vi "Heater Main PID 3.vi"() -> ()   [LabVIEW 2019]
doc: "This example demonstrates how to acquire a continuous amount of data (Waveform) using the DAQ device's internal clock. It also shows how to synchronize two devices for different device families (E Series, S Series, M Series, X Series, DSA, and SC Express), to simultaneously acquire the data.\n\nFor instructions on how to connect your signals to the DAQ device, refer to your device documentation."
uses:
  <vilib>/Utility/error.llb/DialogType.ctl
  <vilib>/DAQmx/read.llb/DAQmx Read (Analog 1D Wfm NChan NSamp).vi
  <vilib>/DAQmx/write.llb/DAQmx Write (Analog DBL 1Chan 1Samp).vi
  <vilib>/DAQmx/create/channels.llb/DAQmx Create Channel (AO-Voltage-Basic).vi
  <vilib>/DAQmx/create/channels.llb/DAQmx Create Channel (AI-Voltage-Basic).vi
panel:
  in  "AI Channel - Heater Shunt":tag
  in  "Channel - Heater V":tag
  in  "Voltage":dbl=1.0 caption="Amplitude"
  in  "Channel config":T1
  in  "error in":errorcluster
  in  "task in":refnum<k21>
  in  "Microhotplate Logger":T2(tab)=enum."Heater config"
  in  "Stop":bool
  in  "Enable logging":bool caption="Enable"
  in  "File config":T3={"Filepath"=path "C:/Users/Administrator/Desktop/DAQ Heater Control/Test data", "Test ID"="test", "PC"="69DTQV2"}
  out "Logging":bool
  in  "Current channel config":T4={"Channel Index"=1, "Shunt resistance"=10.0, "Channel name"="Heater Current"} {"Shunt resistance" format="%.4f"}
  in  "IV channel config":T5={"Voltage channel index"=0, "Current channel index"=2}
  out "IV channel names":T6={"Voltage channel name"="Heater Voltage", "Current channel name"="Heater Current"}
  in  "TCR config":T7={"TCR1"=0.00205, "TCR2"=3e-07, "TRH"=0.766, "TRM"=0.928} {"TRM" format="%.3f"; "TRH" format="%.3f"; "TCR2" format="%.2e"; "TCR1" format="%.2e"}
  in  "Ramb config":cluster{"Tamb":dbl, "Ramb":dbl}={"Tamb"=25.0, "Ramb"=4.84} {"Ramb" format="%.3f"; "Tamb" format="%.3f"}
  out "Shunt channel name":string="Heater Shunt"
  out "PID output":dbl=1.0
  out "PID input":dbl
  in  "Setpoint":i32=2
  in  "Increment":dbl format="%.4f"
  out "Overrange":bool
  out "Heater shunt":dynamicdata(graph)=[{"t0"=timestamp(3680167673.7458043 s since 1904-01-01), "dt"=0.001, "Y"=[0.23414337637449473], "attributes"=variant("NI_ChannelName"=variant(string "Heater Voltage (DC Voltage)"), "NI_OriginalChannelName"=variant(string "Heater Voltage"), "NI_UnitDescription"=variant(string "Volts"))}, {"t0"=timestamp(3680167673.7458158 s since 1904-01-01), "dt"=0.001, "Y"=[0.4133136878458651], "attributes"=variant("NI_ChannelName"=variant(string "Heater Shunt (DC Voltage)"), "NI_OriginalChannelName"=variant(string "Heater Shunt"), "NI_UnitDescription"=variant(string "Volts"))}, {"t0"=timestamp(3680167673.7458158 s since 1904-01-01), "dt"=0.001, "Y"=[0.04133136878458673], "attributes"=variant("NI_ChannelName"=variant(string "Heater Current (DC Voltage)"), "NI_OriginalChannelName"=variant(string "Heater Current"), "NI_UnitDescription"=variant(string "A"))}, {"t0"=timestamp(3680167673.7458043 s since 1904-01-01), "dt"=0.001, "Y"=[5.665028733285053], "attributes"=variant("NI_ChannelName"=variant(string "Heater Resistance (DC Voltage)"), "NI_OriginalChannelName"=variant(string "Heater Resistance"), "NI_UnitDescription"=variant(string "Ohms"))}, {"t0"=timestamp(3680167673.7458043 s since 1904-01-01), "dt"=0.001, "Y"=[0.009677466447099818], "attributes"=variant("NI_ChannelName"=variant(string "Heater Power (DC Voltage)"), "NI_OriginalChannelName"=variant(string "Heater Power"), "NI_UnitDescription"=variant(string "Ohms"))}, {"t0"=timestamp(3680167673.7458043 s since 1904-01-01), "dt"=0.001, "Y"=[124.29416718343353], "attributes"=variant("NI_ChannelName"=variant(string "Heater Temp (DC Voltage)"), "NI_OriginalChannelName"=variant(string "Heater Temp"), "NI_UnitDescription"=variant(string "degC"))}]
  out "Heater temperature":dynamicdata(graph)=[{"t0"=timestamp(3680167673.7458043 s since 1904-01-01), "dt"=0.001, "Y"=[0.23414337637449473], "attributes"=variant("NI_ChannelName"=variant(string "Heater Voltage (DC Voltage)"), "NI_OriginalChannelName"=variant(string "Heater Voltage"), "NI_UnitDescription"=variant(string "Volts"))}, {"t0"=timestamp(3680167673.7458158 s since 1904-01-01), "dt"=0.001, "Y"=[0.4133136878458651], "attributes"=variant("NI_ChannelName"=variant(string "Heater Shunt (DC Voltage)"), "NI_OriginalChannelName"=variant(string "Heater Shunt"), "NI_UnitDescription"=variant(string "Volts"))}, {"t0"=timestamp(3680167673.7458158 s since 1904-01-01), "dt"=0.001, "Y"=[0.04133136878458673], "attributes"=variant("NI_ChannelName"=variant(string "Heater Current (DC Voltage)"), "NI_OriginalChannelName"=variant(string "Heater Current"), "NI_UnitDescription"=variant(string "A"))}, {"t0"=timestamp(3680167673.7458043 s since 1904-01-01), "dt"=0.001, "Y"=[5.665028733285053], "attributes"=variant("NI_ChannelName"=variant(string "Heater Resistance (DC Voltage)"), "NI_OriginalChannelName"=variant(string "Heater Resistance"), "NI_UnitDescription"=variant(string "Ohms"))}, {"t0"=timestamp(3680167673.7458043 s since 1904-01-01), "dt"=0.001, "Y"=[0.009677466447099818], "attributes"=variant("NI_ChannelName"=variant(string "Heater Power (DC Voltage)"), "NI_OriginalChannelName"=variant(string "Heater Power"), "NI_UnitDescription"=variant(string "Ohms"))}, {"t0"=timestamp(3680167673.7458043 s since 1904-01-01), "dt"=0.001, "Y"=[124.29416718343353], "attributes"=variant("NI_ChannelName"=variant(string "Heater Temp (DC Voltage)"), "NI_OriginalChannelName"=variant(string "Heater Temp"), "NI_UnitDescription"=variant(string "degC"))}]
  out "Heater current":dynamicdata(graph)=[{"t0"=timestamp(3680167673.7458043 s since 1904-01-01), "dt"=0.001, "Y"=[0.23414337637449473], "attributes"=variant("NI_ChannelName"=variant(string "Heater Voltage (DC Voltage)"), "NI_OriginalChannelName"=variant(string "Heater Voltage"), "NI_UnitDescription"=variant(string "Volts"))}, {"t0"=timestamp(3680167673.7458158 s since 1904-01-01), "dt"=0.001, "Y"=[0.4133136878458651], "attributes"=variant("NI_ChannelName"=variant(string "Heater Shunt (DC Voltage)"), "NI_OriginalChannelName"=variant(string "Heater Shunt"), "NI_UnitDescription"=variant(string "Volts"))}, {"t0"=timestamp(3680167673.7458158 s since 1904-01-01), "dt"=0.001, "Y"=[0.04133136878458673], "attributes"=variant("NI_ChannelName"=variant(string "Heater Current (DC Voltage)"), "NI_OriginalChannelName"=variant(string "Heater Current"), "NI_UnitDescription"=variant(string "A"))}, {"t0"=timestamp(3680167673.7458043 s since 1904-01-01), "dt"=0.001, "Y"=[5.665028733285053], "attributes"=variant("NI_ChannelName"=variant(string "Heater Resistance (DC Voltage)"), "NI_OriginalChannelName"=variant(string "Heater Resistance"), "NI_UnitDescription"=variant(string "Ohms"))}, {"t0"=timestamp(3680167673.7458043 s since 1904-01-01), "dt"=0.001, "Y"=[0.009677466447099818], "attributes"=variant("NI_ChannelName"=variant(string "Heater Power (DC Voltage)"), "NI_OriginalChannelName"=variant(string "Heater Power"), "NI_UnitDescription"=variant(string "Ohms"))}, {"t0"=timestamp(3680167673.7458043 s since 1904-01-01), "dt"=0.001, "Y"=[124.29416718343353], "attributes"=variant("NI_ChannelName"=variant(string "Heater Temp (DC Voltage)"), "NI_OriginalChannelName"=variant(string "Heater Temp"), "NI_UnitDescription"=variant(string "degC"))}]
  out "Heater voltage":dynamicdata(graph)=[{"t0"=timestamp(3680167673.7458043 s since 1904-01-01), "dt"=0.001, "Y"=[0.23414337637449473], "attributes"=variant("NI_ChannelName"=variant(string "Heater Voltage (DC Voltage)"), "NI_OriginalChannelName"=variant(string "Heater Voltage"), "NI_UnitDescription"=variant(string "Volts"))}, {"t0"=timestamp(3680167673.7458158 s since 1904-01-01), "dt"=0.001, "Y"=[0.4133136878458651], "attributes"=variant("NI_ChannelName"=variant(string "Heater Shunt (DC Voltage)"), "NI_OriginalChannelName"=variant(string "Heater Shunt"), "NI_UnitDescription"=variant(string "Volts"))}, {"t0"=timestamp(3680167673.7458158 s since 1904-01-01), "dt"=0.001, "Y"=[0.04133136878458673], "attributes"=variant("NI_ChannelName"=variant(string "Heater Current (DC Voltage)"), "NI_OriginalChannelName"=variant(string "Heater Current"), "NI_UnitDescription"=variant(string "A"))}, {"t0"=timestamp(3680167673.7458043 s since 1904-01-01), "dt"=0.001, "Y"=[5.665028733285053], "attributes"=variant("NI_ChannelName"=variant(string "Heater Resistance (DC Voltage)"), "NI_OriginalChannelName"=variant(string "Heater Resistance"), "NI_UnitDescription"=variant(string "Ohms"))}, {"t0"=timestamp(3680167673.7458043 s since 1904-01-01), "dt"=0.001, "Y"=[0.009677466447099818], "attributes"=variant("NI_ChannelName"=variant(string "Heater Power (DC Voltage)"), "NI_OriginalChannelName"=variant(string "Heater Power"), "NI_UnitDescription"=variant(string "Ohms"))}, {"t0"=timestamp(3680167673.7458043 s since 1904-01-01), "dt"=0.001, "Y"=[124.29416718343353], "attributes"=variant("NI_ChannelName"=variant(string "Heater Temp (DC Voltage)"), "NI_OriginalChannelName"=variant(string "Heater Temp"), "NI_UnitDescription"=variant(string "degC"))}]
  out "Heater resistance":dynamicdata(graph)=[{"t0"=timestamp(3680167673.7458043 s since 1904-01-01), "dt"=0.001, "Y"=[0.23414337637449473], "attributes"=variant("NI_ChannelName"=variant(string "Heater Voltage (DC Voltage)"), "NI_OriginalChannelName"=variant(string "Heater Voltage"), "NI_UnitDescription"=variant(string "Volts"))}, {"t0"=timestamp(3680167673.7458158 s since 1904-01-01), "dt"=0.001, "Y"=[0.4133136878458651], "attributes"=variant("NI_ChannelName"=variant(string "Heater Shunt (DC Voltage)"), "NI_OriginalChannelName"=variant(string "Heater Shunt"), "NI_UnitDescription"=variant(string "Volts"))}, {"t0"=timestamp(3680167673.7458158 s since 1904-01-01), "dt"=0.001, "Y"=[0.04133136878458673], "attributes"=variant("NI_ChannelName"=variant(string "Heater Current (DC Voltage)"), "NI_OriginalChannelName"=variant(string "Heater Current"), "NI_UnitDescription"=variant(string "A"))}, {"t0"=timestamp(3680167673.7458043 s since 1904-01-01), "dt"=0.001, "Y"=[5.665028733285053], "attributes"=variant("NI_ChannelName"=variant(string "Heater Resistance (DC Voltage)"), "NI_OriginalChannelName"=variant(string "Heater Resistance"), "NI_UnitDescription"=variant(string "Ohms"))}, {"t0"=timestamp(3680167673.7458043 s since 1904-01-01), "dt"=0.001, "Y"=[0.009677466447099818], "attributes"=variant("NI_ChannelName"=variant(string "Heater Power (DC Voltage)"), "NI_OriginalChannelName"=variant(string "Heater Power"), "NI_UnitDescription"=variant(string "Ohms"))}, {"t0"=timestamp(3680167673.7458043 s since 1904-01-01), "dt"=0.001, "Y"=[124.29416718343353], "attributes"=variant("NI_ChannelName"=variant(string "Heater Temp (DC Voltage)"), "NI_OriginalChannelName"=variant(string "Heater Temp"), "NI_UnitDescription"=variant(string "degC"))}]
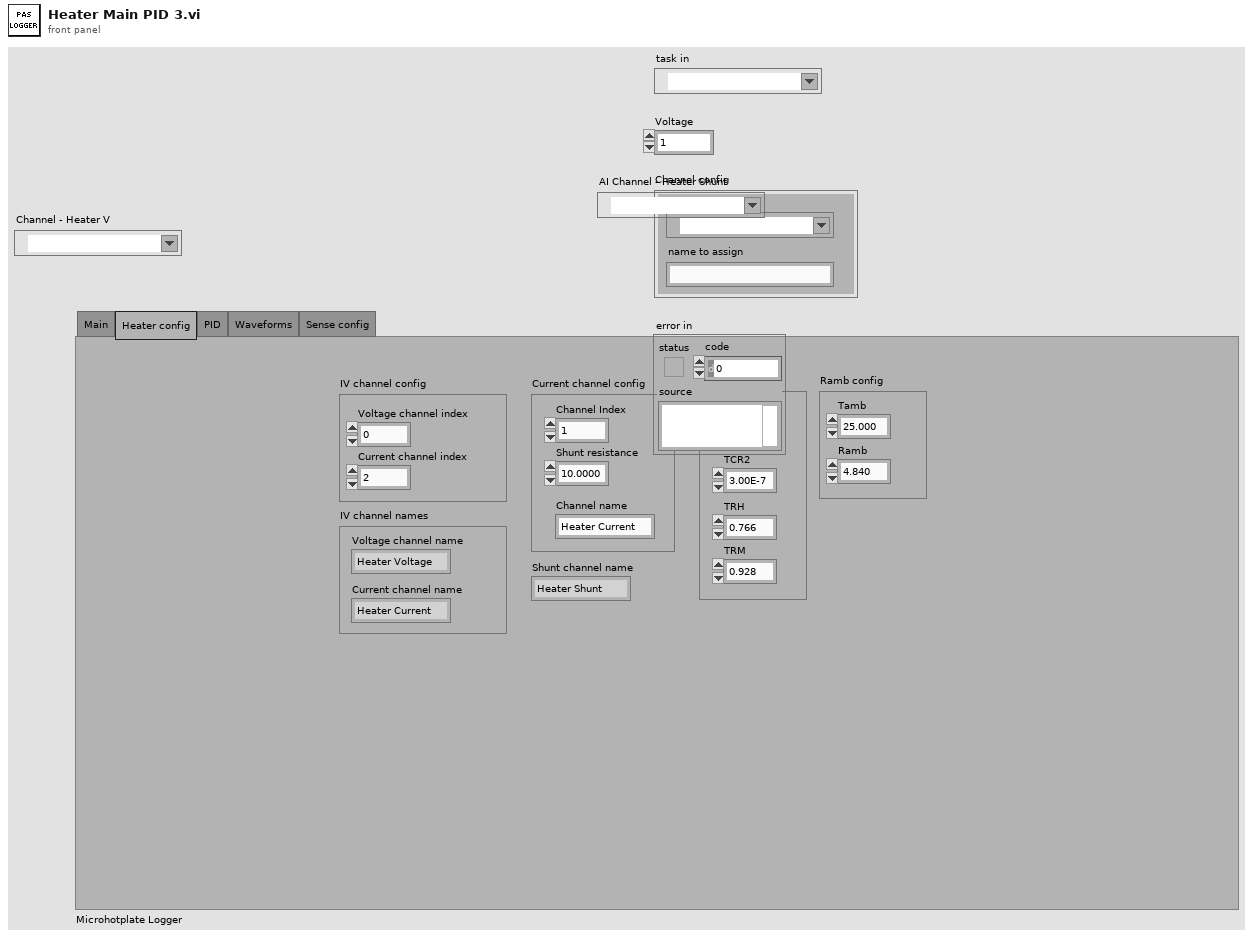
[diagram p1: front panel]
types:
  T1 = cluster{"Output channel":tag, "name to assign":string}
  T2 = enum32{"Main", "Heater config", "PID", "Waveforms", "Sense config"}
  T3 = cluster{"Filepath":path, "Test ID":string, "PC":string}
  T4 = cluster{"Channel Index":i32, "Shunt resistance":dbl, "Channel name":string}
  T5 = cluster{"Voltage channel index":i32, "Current channel index":i32}
  T6 = cluster{"Voltage channel name":string, "Current channel name":string}
  T7 = cluster{"TCR1":dbl, "TCR2":dbl, "TRH":dbl, "TRM":dbl}
  T8 = typedef "DialogType.ctl" = u16
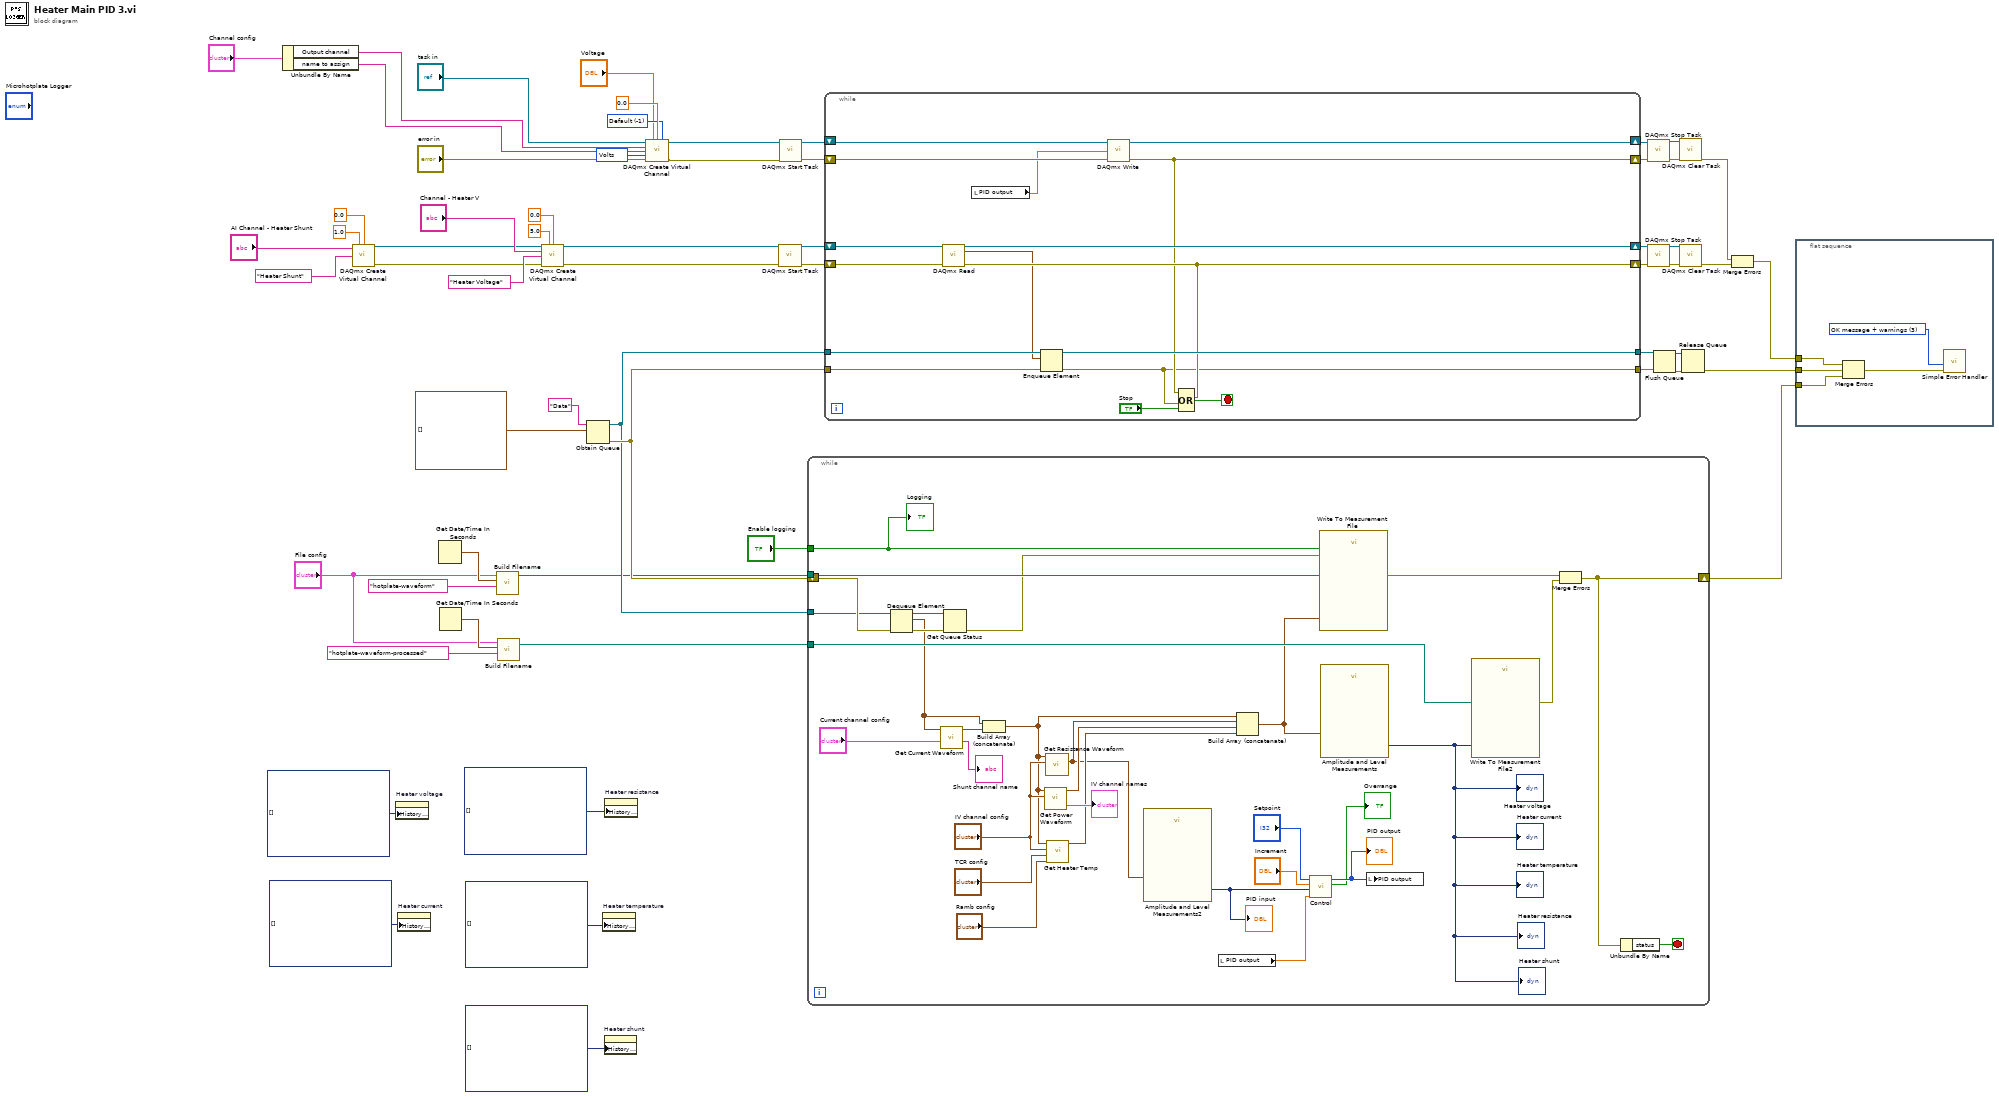
[diagram p0: block diagram]
diagram:
  w17 = 10348 items=["Volts"=10348, "From Custom Scale"=10065] ("units")
  w18 = -1 items=["Default"=-1, "RSE"=10083, "Differential"=10106, "Pseudodifferential"=12529] ("output terminal configuration")
  n1 = Unbundle By Name("Channel config") -> ("Output channel"=w19:tag, "name to assign"=w5:string)
  n2 = call-poly <vilib>:"DAQmx Create Virtual Channel.vi"("maximum value"=1.0 ("maximum value 2"), "minimum value"=0.0 ("minimum value 2"), "physical channels"="AI Channel - Heater Shunt", "name to assign"="Heater Shunt") -> ("task out"=w1:refnum<k21>, "error out"=w7:errorcluster)  [unwired: 10 in]
  n3 = property on="Heater voltage" class="WFChart (strict)"("History Data"=dynamicdata[] []) -> ()  [unwired: 2 in, 2 out]
  n4 = property on="Heater current" class="WFChart (strict)"("History Data"=dynamicdata[] []) -> ()  [unwired: 2 in, 2 out]
  n5 = Get Date/Time In Seconds() -> (seconds since 1Jan1904=w33:timestamp)
  n6 = Get Date/Time In Seconds() -> (seconds since 1Jan1904=w31:timestamp)
  n7 = call "Build Filename.vi"("Test type"="hotplate-waveform" ("File type"), "time stamp"=w33, "File config"="File config") -> ("appended path"=w35:path)  [unwired: 8 in]
  n8 = call "Build Filename.vi"("Test type"="hotplate-waveform-processed" ("File type"), "time stamp"=w31, "File config"="File config") -> ("appended path"=w30:path)  [unwired: 8 in]
  n9 = call-poly <vilib>:"DAQmx Create Virtual Channel.vi"("task in"=w1, "maximum value"=5.0, "minimum value"=0.0, "physical channels"="Channel - Heater V", "name to assign"="Heater Voltage", "error in"=w7) -> ("task out"=w13:refnum<k21>, "error out"=w12:errorcluster)  [unwired: 8 in]
  n10 = Obtain Queue(name (unnamed)="Data" ("名前（名前なし）"), element data type=waveform(dbl)[] [] ("data")) -> (queue out=w39:refnum<queue>, error out=w40:errorcluster)  [unwired: 3 in, 1 out]
  n11 = property on="Heater temperature" class="WFChart (strict)"("History Data"=dynamicdata[] []) -> ()  [unwired: 2 in, 2 out]
  n12 = property on="Heater shunt" class="WFChart (strict)"("History Data"=dynamicdata[] []) -> ()  [unwired: 2 in, 2 out]
  n13 = property on="Heater resistance" class="WFChart (strict)"("History Data"=dynamicdata[] []) -> ()  [unwired: 2 in, 2 out]
  n14 = call-poly <vilib>:"DAQmx Create Virtual Channel.vi"("task in"="task in", "maximum value"="Voltage", "minimum value"=0.0, "output terminal configuration"=w18, "physical channels"=w19, "name to assign"=w5, "units"=w17, "error in"="error in") -> ("task out"=w14:refnum<k21>, "error out"=w15:errorcluster)  [unwired: 6 in]
  n15 = call <vilib>:"DAQmx Start Task.vi"("task/channels in"=w13, "error in"=w12) -> ("task out"=w48:refnum<k21>, "error out"=w49:errorcluster)  [unwired: 12 in]
  n16 = call <vilib>:"DAQmx Start Task.vi"("task/channels in"=w14, "error in"=w15) -> ("task out"=w50:refnum<k21>, "error out"=w51:errorcluster)  [unwired: 12 in]
  n17 = while {
    tunnel: w39 -> [w92]
    shift-right: [w85] -> w38
    shift-left: w40 -> [w93]
    tunnel: w35 -> [w91]
    tunnel: "Enable logging" -> [w87]
    tunnel: w30 -> [w82]
    stop <- w84 stop-if-true
    n18 = Dequeue Element(queue=w92, error in (no error)=w93) -> (queue out=w89:refnum<queue>, element=w73:waveform(dbl)[], error out=w90:errorcluster)  [unwired: 1 in, 1 out]
    n19 = call "Get Current Waveform.vi"("Config"="Current channel config", "array"=w73) -> ("Channel name"=→"Shunt channel name":string, "Current waveform out"=w79:waveform(dbl))  [unwired: 8 in]
    n20 = Get Queue Status(queue=w89, error in (no error)=w90) -> (error out=w88:errorcluster)  [unwired: 1 in, 7 out]
    n21 = Build Array (concatenate)(w73, w79) -> (w71:waveform(dbl)[])
    n22 = call "Get Power Waveform.vi"("Channel config"="IV channel config", "array"=w71) -> ("Power waveform out"=w74:waveform(dbl), "Channel names"=→"IV channel names":T6)  [unwired: 8 in]
    n23 = call "Get Resistance Waveform.vi"("Channel config"="IV channel config", "array"=w71) -> ("Resistance waveform out"=w64:waveform(dbl))  [unwired: 8 in, 1 out]
    n24 = call "Get Heater Temp.vi"("Ramb config"="Ramb config", "TCR config"="TCR config", "Channel config"="IV channel config", "array"=w71) -> ("waveform out"=w69:waveform(dbl))  [unwired: 6 in, 1 out]
    n25 = call "Amplitude and Level Measurements2"("Signals"=w64) -> ("Mean (DC)"=w63:dynamicdata)  [unwired: 13 in, 1 out]
    "PID input" <- w63
    n26 = local read "PID output"() -> (w65:dbl)
    n27 = Build Array (concatenate)(w71, w64, w74, w69) -> (w81:waveform(dbl)[])
    n28 = call "Control.vi"("Control in"=w65, "Sense"=w63, "Increment"="Increment", "Setpoint"="Setpoint") -> ("Overrange"=→"Overrange":bool, "Control out"=w66:i32)  [unwired: 6 in]
    "PID output" <- w66
    n29 = call "Write To Measurement File"("Signals"=w81, "Enable"=w87, "error in (no error)"=w88, "Filename"=w91) -> ("error out"=w86:errorcluster)  [unwired: 13 in, 2 out]
    n30 = call "Amplitude and Level Measurements"("Signals"=w81) -> ("Mean (DC)"=w72:dynamicdata)  [unwired: 13 in, 1 out]
    "Heater voltage" <- w72
    "Heater current" <- w72
    "Heater temperature" <- w72
    "Heater resistance" <- w72
    "Heater shunt" <- w72
    n31 = local write "PID output"(w66) -> ()
    n32 = call "Write To Measurement File2"("Signals"=w72, "Filename"=w82) -> ("error out"=w83:errorcluster)  [unwired: 15 in, 2 out]
    n33 = Merge Errors(w86, w83) -> (w85:errorcluster)
    n34 = Unbundle By Name(w85) -> ("status"=w84:bool)
    "Logging" <- w87
  }
  n35 = while {
    shift-right: [w98] -> w60
    shift-left: w51 -> [w99]
    shift-right: [w101] -> w56
    shift-left: w49 -> [w108]
    shift-right: [w96] -> w61
    shift-left: w50 -> [w97]
    shift-right: [w107] -> w57
    shift-left: w48 -> [w109]
    tunnel: [w105] -> w45
    tunnel: [w95] -> w44
    tunnel: w39 -> [w104]
    tunnel: w40 -> [w103]
    stop <- w110 stop-if-true
    n36 = call-poly <vilib>:"DAQmx Read.vi"("task/channels in"=w109, "error in"=w108) -> ("task out"=w107:refnum<k21>, "data"=w100:waveform(dbl)[], "number of samples per channel"=w106:i32, "error out"=w101:errorcluster)  [unwired: 10 in]
    n37 = local read "PID output"() -> (w94:dbl)
    n38 = Enqueue Element(queue=w104, element=w100, error in (no error)=w103) -> (queue out=w105:refnum<queue>, error out=w95:errorcluster)  [unwired: 1 in, 1 out]
    n39 = call-poly <vilib>:"DAQmx Write.vi"("task/channels in"=w97, "data"=w94, "error in"=w99) -> ("task out"=w96:refnum<k21>, "error out"=w98:errorcluster)  [unwired: 10 in, 1 out]
    n40 = Compound Arithmetic op=OR(w98, w101, w95, "Stop") -> (w110:bool)
  }
  n41 = call <vilib>:"DAQmx Stop Task.vi"("task/channels in"=w61, "error in"=w60) -> ("task out"=w58:refnum<k21>, "error out"=w59:errorcluster)  [unwired: 12 in]
  n42 = call <vilib>:"DAQmx Stop Task.vi"("task/channels in"=w57, "error in"=w56) -> ("task out"=w54:refnum<k21>, "error out"=w55:errorcluster)  [unwired: 12 in]
  n43 = Flush Queue(queue=w45, error in (no error)=w44) -> (queue out=w46:refnum<queue>, error out=w47:errorcluster)  [unwired: 1 out]
  n44 = call <vilib>:"DAQmx Clear Task.vi"("task in"=w58, "error in"=w59) -> ("error out"=w53:errorcluster)  [unwired: 13 in]
  n45 = call <vilib>:"DAQmx Clear Task.vi"("task in"=w54, "error in"=w55) -> ("error out"=w52:errorcluster)  [unwired: 13 in]
  n46 = Release Queue(queue=w46, error in (no error)=w47) -> (error out=w42:errorcluster)  [unwired: 1 in, 2 out]
  n47 = Merge Errors(w53, w52) -> (w43:errorcluster)
  n48 = flat-sequence {
    tunnel: w43 -> [w115]
    tunnel: w42 -> [w114]
    tunnel: w38 -> [w111]
    frame #0 {
      w113 = T8 3 items=["no dialog", "OK message", "continue or stop message", "OK message + warnings", "continue/stop + warnings"] ("type of dialog (OK msg:1)")
      n49 = Merge Errors(w115, w114, w111) -> (w112:errorcluster)
      n50 = call <vilib>:"Simple Error Handler.vi"("type of dialog (OK msg:1)"=w113, "error in (no error)"=w112) -> ()  [unwired: 3 in, 5 out]
    }
  }
